vi "Digital_Input.vi"() -> ()   [LabVIEW 2018]
panel:
  out "data":bool[](array[boolean]) caption="데이터"
  in  "정지":bool
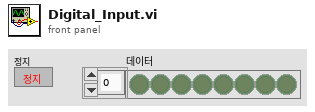
[diagram p1: front panel]
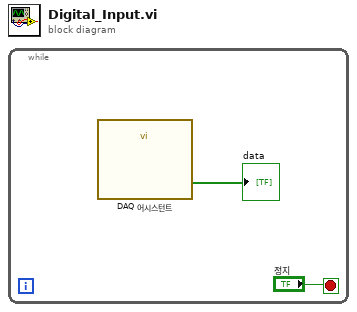
[diagram p0: block diagram]
diagram:
  n1 = while {
    stop <- "정지" stop-if-true
    n2 = call "DAQ 어시스턴트"() -> ("data"=→"data":bool[])  [unwired: 17 in, 2 out]
  }
